vi "Chrg_Dschrg_nodaq.vi"(0 "Mod #":enum16{"0", "1", "2", "3"}(ring), 1 "Logical Instrument Number":u32=1, 3 "PS type":enum16{"ITECH", "NHR"}(ring), 4 "PS VISA in":refnum<visa-resource-name>, 5 "PS error in":errorcluster caption="PS error in (no error)", 6 "CyclePath":path=path "C:/Users/ga11/Desktop/VI/results/3PtestCharge.lvm" caption="Filename", 7 "Battery Type":T1(ring), 8 "Charge/discharge":enum8{"Charge", "Discharge"}(ring), 9 "Charge/Discharge Voltage Setpoint":dbl format="%#.6g", 11 "Current Setpoint":dbl format="%#.6g", 13 "Current Cutoff":dbl) -> (14 "PS VISA out":refnum<visa-resource-name>, 19 "PS error out":errorcluster)   [LabVIEW 2020]
uses:
  vi.lib/Utility/TradDaqScaling.llb/Convert Strain Gauge Reading (scaler).vi
  Drivers-NHR-9200/NHR/Public/Data/Read (Ave Current).vi
  Drivers-NHR-9200/NHR/Public/Data/Low Level/Fetch (Ave Voltage).vi
  Drivers-Essentials/NH Research Regenerative Test Series.lvlib
  Drivers-IT-M3400/IT-M3400.lvlib
panel:
  out "StrainGauge 2":dbl format="%.10f"
  out "Thermocouple 2":dbl format="%.2f"
  out "StrainGauge 1":dbl format="%.10f"
  out "Thermocouple 1":dbl format="%.2f"
  out "StrainGauge 3":dbl format="%.10f"
  out "Thermocouple 3":dbl format="%.2f"
  out "StrainGauge":dbl format="%.10f"
  out "Thermocouple":dbl format="%.2f"
  out "Read Ave Current (A)":dbl
  out "Read Ave Voltage (V)":dbl
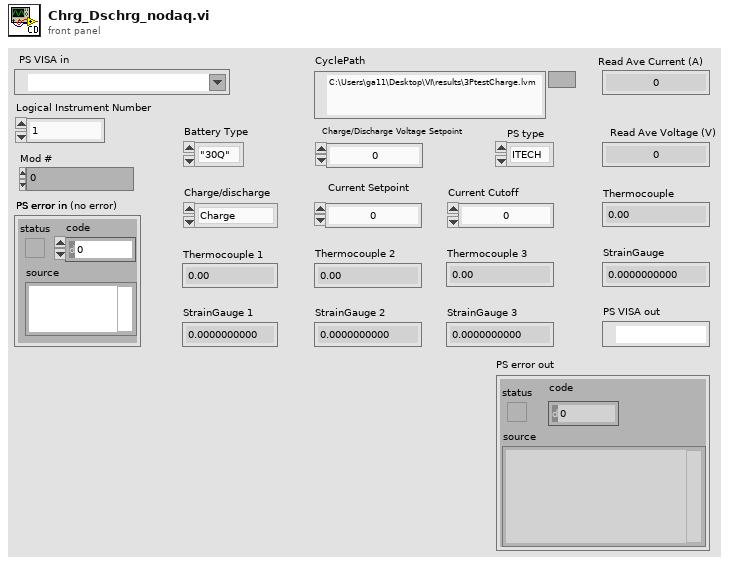
[diagram p1: front panel]
types:
  T1 = enum16{"\"30Q\"", "\"40T\"", "\"2P30Q\"", "\"3P30Q\"", "\"Nissan Leaf\""}
  T2 = cluster{"Min Voltage (V)":dbl, "Min Voltage Time (s)":dbl, "Max Voltage (V)":dbl, "Max Voltage Time (s)":dbl, "Max Sink Current (A)":dbl, "Max Sink Current Time (s)":dbl, "Max Source Current (A)":dbl, "Max Source Current Time (s)":dbl, "Max Sink Power (W)":dbl, "Max Sink Power Time (s)":dbl, "Max Source Power (W)":dbl, "Max Source Power Time (s)":dbl}
  T3 = cluster{"Voltage Enabled":bool, "Current Enabled":bool, "Power Enabled":bool, "Resistance Enabled":bool}
  T4 = cluster{"Baud Rate":u32, "Parity":u16, "Data Bits":u16, "Stop Bits":u16, "Flow Control":u16}
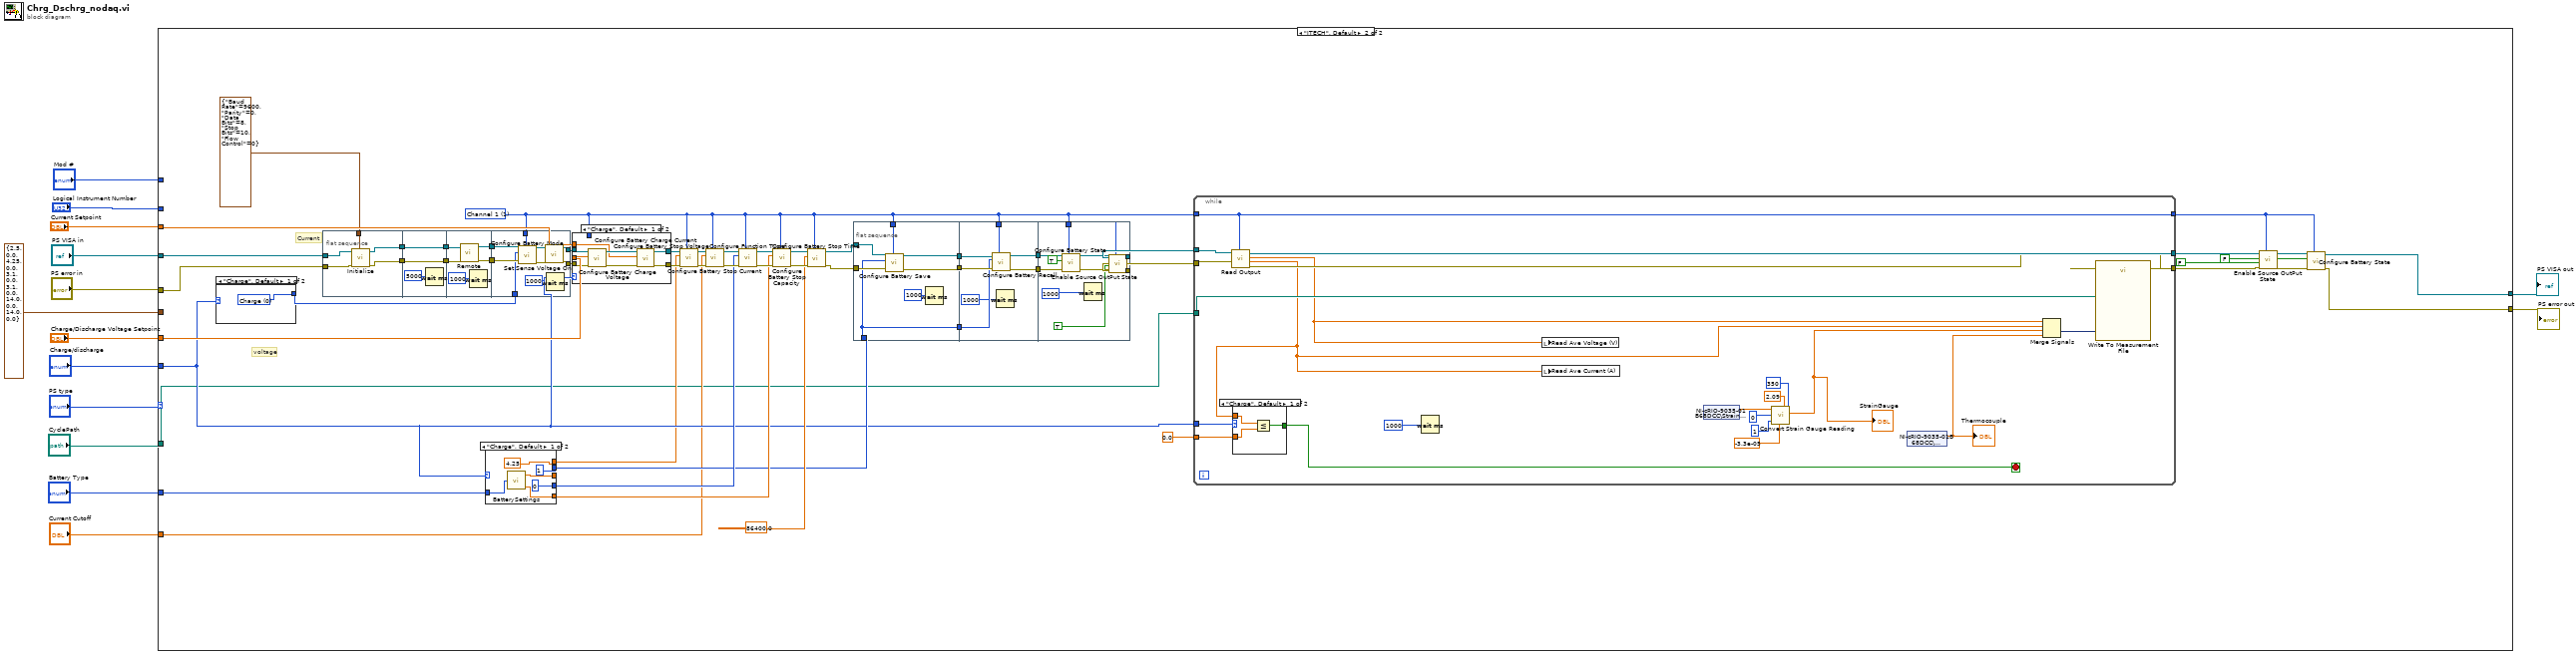
[diagram p0: block diagram]
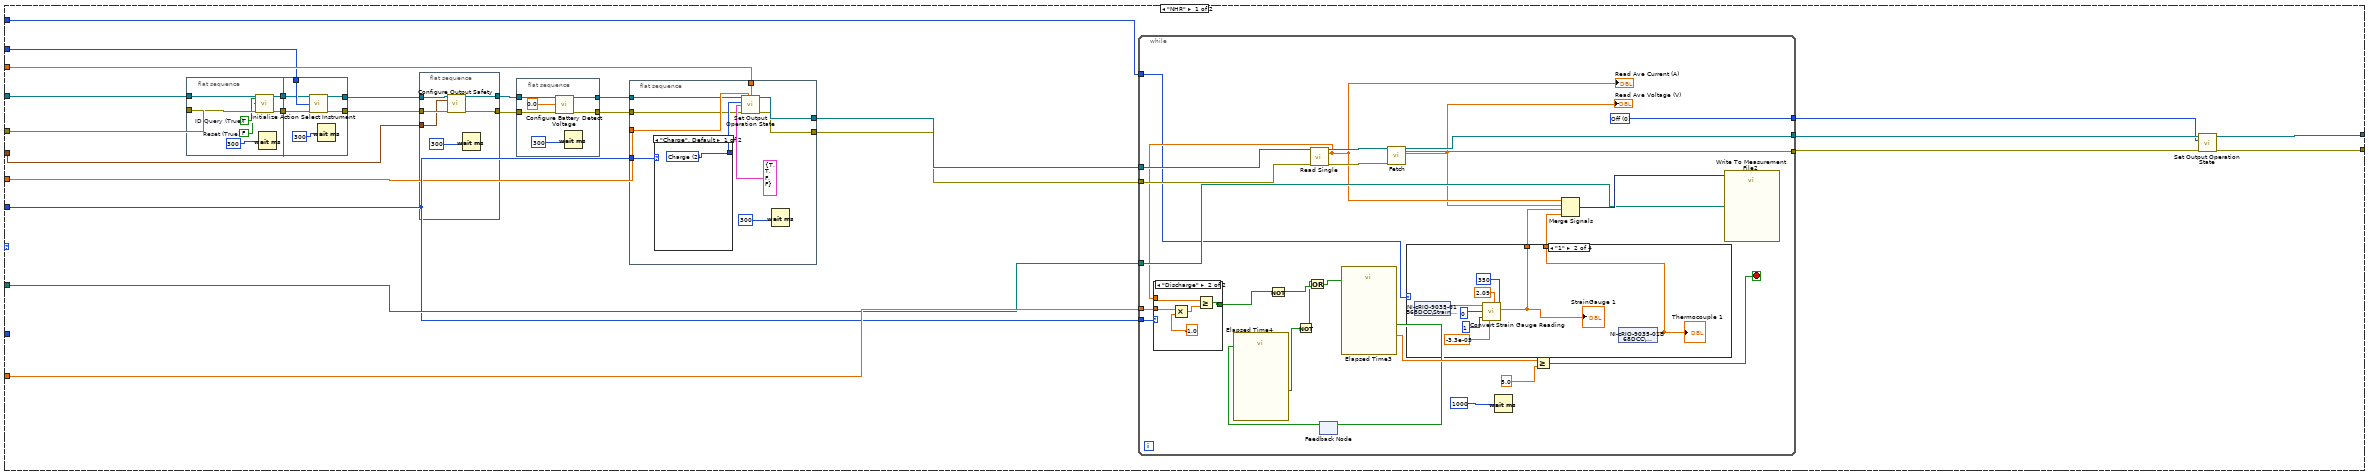
[diagram p2: hidden frame]
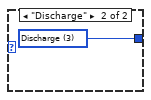
[diagram p3: hidden frame]
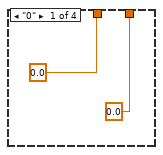
[diagram p4: hidden frame]
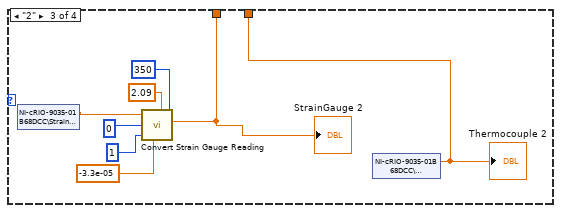
[diagram p5: hidden frame]
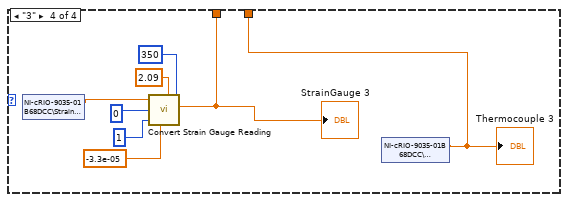
[diagram p6: hidden frame]
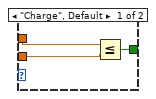
[diagram p7: hidden frame]
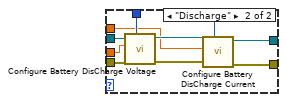
[diagram p8: hidden frame]
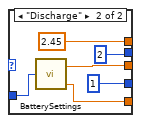
[diagram p9: hidden frame]
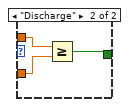
[diagram p10: hidden frame]
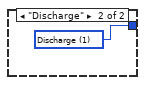
[diagram p11: hidden frame]
diagram:
  n1 = case shown="\"ITECH\", Default" "PS type" {
    tunnel: "Charge/Discharge Voltage Setpoint" -> [w29 w175]
    tunnel: "Current Setpoint" -> [w30 w173]
    tunnel: "Current Cutoff" -> [w37 w143]
    tunnel: "CyclePath" -> [w36 w141]
    tunnel: "PS VISA in" -> [w21 w154]
    tunnel: "PS error in" -> [w20 w153]
    tunnel: [w35 w140] -> w4
    tunnel: [w34 w174] -> w8
    tunnel: "Charge/discharge" -> [w31 w144]
    tunnel: "Battery Type" -> [_ w172]
    tunnel: "Mod #" -> [w27 _]
    tunnel: T2 {"Min Voltage (V)"=2.5, "Min Voltage Time (s)"=0.0, "Max Voltage (V)"=4.25, "Max Voltage Time (s)"=0.0, "Max Sink Current (A)"=3.1, "Max Sink Current Time (s)"=0.0, "Max Source Current (A)"=3.1, "Max Source Current Time (s)"=0.0, "Max Sink Power (W)"=14.0, "Max Sink Power Time (s)"=0.0, "Max Source Power (W)"=14.0, "Max Source Power Time (s)"=0.0} ("Output Safety") -> [w22 _]
    tunnel: "Logical Instrument Number" -> [w19 _]
    frame "NHR" {
      n2 = flat-sequence {
        tunnel: w21 -> [w46]
        tunnel: w20 -> [w45]
        tunnel: [w42] -> w16
        tunnel: [w41] -> w15
        tunnel: w19 -> [w52]
        tunnel: [w51] -> w18
        tunnel: [w50] -> w17
        tunnel: w16 -> [w49]
        tunnel: w15 -> [w48]
        frame #0 {
          w43 = FALSE  # Reset (True)
          w44 = TRUE  # ID Query (True)
          n3 = call "Initialize.vi"("VISA resource name"=w46, "ID Query (True)"=w44, "Reset (True)"=w43, "error in (no error)"=w45) -> ("VISA resource name out"=w41:refnum<visa-resource-name>, "error out"=w42:errorcluster)  [unwired: 10 in]
          n4 = Wait (ms)(milliseconds to wait=300) -> ()  [unwired: 1 out]
        }
        frame #1 {
          n5 = call "Action Select Instrument.vi"("VISA resource name"=w48, "Logical Instrument Number"=w52, "error in (no error)"=w49) -> ("VISA resource name out"=w51:refnum<visa-resource-name>, "error out"=w50:errorcluster)  [unwired: 11 in]
          n6 = Wait (ms)(milliseconds to wait=300) -> ()  [unwired: 1 out]
        }
      }
      n7 = flat-sequence {
        tunnel: w18 -> [w63]
        tunnel: w17 -> [w62]
        tunnel: [w61] -> w25
        tunnel: [w60] -> w26
        tunnel: w22 -> [w59]
        frame #0 {
          n8 = call "Configure Output Safety.vi"("VISA resource name"=w63, "Output Safety"=w59, "error in (no error)"=w62) -> ("VISA resource name out"=w60:refnum<visa-resource-name>, "error out"=w61:errorcluster)  [unwired: 11 in]
          n9 = Wait (ms)(milliseconds to wait=300) -> ()  [unwired: 1 out]
        }
      }
      n10 = flat-sequence {
        tunnel: w26 -> [w56]
        tunnel: w25 -> [w55]
        tunnel: [w54] -> w24
        tunnel: [w53] -> w23
        frame #0 {
          n11 = call "Configure Battery Detect Voltage.vi"("VISA resource name"=w56, "Battery Detect Voltage (0V)"=0.0, "error in (no error)"=w55) -> ("VISA resource name out"=w53:refnum<visa-resource-name>, "error out"=w54:errorcluster)  [unwired: 11 in]
          n12 = Wait (ms)(milliseconds to wait=300) -> ()  [unwired: 1 out]
        }
      }
      n13 = flat-sequence {
        tunnel: [w74] -> w39
        tunnel: [w73] -> w38
        tunnel: w31 -> [w71]
        tunnel: w30 -> [w70]
        tunnel: w29 -> [w69]
        tunnel: w24 -> [w66]
        tunnel: w23 -> [w65]
        frame #0 {
          n14 = case shown="\"Charge\", Default" w71 {
            tunnel: [w75 w76] -> w72
            frame "Charge", Default {
              w75 = 2 items=["Off", "Standby", "Charge", "Discharge", "Battery"] ("Mode (0: Off)")
            }
            frame "Discharge" {
              w76 = 3 items=["Off", "Standby", "Charge", "Discharge", "Battery"] ("Mode (0: Off)")
            }
          }
          n15 = call "Set Output Operation State.vi"("VISA resource name"=w65, "Voltage Setpoint (0 V)"=w69, "Current Setpoint (0 A)"=w70, "Mode (0: Off)"=w72, "Enable"=T3 {"Voltage Enabled"=TRUE, "Current Enabled"=TRUE, "Power Enabled"=FALSE, "Resistance Enabled"=FALSE}, "error in (no error)"=w66, "Power Setpoint (0 W)"=w69) -> ("VISA resource name out"=w74:refnum<visa-resource-name>, "error out"=w73:errorcluster)  [unwired: 7 in]
          n16 = Wait (ms)(milliseconds to wait=300) -> ()  [unwired: 1 out]
        }
      }
      n17 = while {
        tunnel: w39 -> [w101]
        tunnel: w38 -> [w100]
        tunnel: w37 -> [w85]
        tunnel: w36 -> [w88]
        tunnel: [w87] -> w33
        tunnel: [w86] -> w32
        tunnel: w31 -> [w84]
        tunnel: w27 -> [w78]
        tunnel: [w77] -> w28
        stop <- w91 stop-if-true
        w77 = 0 items=["Off", "Standby", "Charge", "Discharge", "Battery"] ("Mode (0: Off)")
        n18 = call-poly "Read Single.vi"("VISA resource name"=w101, "error in (no error)"=w100) -> ("VISA resource name out"=w102:refnum<visa-resource-name>, "Ave Current (A)"=w83:dbl, "error out"=w103:errorcluster)  [unwired: 11 in]
        "Read Ave Current (A)" <- w83
        n19 = case shown="\"Discharge\"" w84 {
          tunnel: w85 -> [w130 w136]
          tunnel: w83 -> [w132 w134]
          tunnel: [w131 w133] -> w82
          frame "Charge", Default {
            n20 = Less Or Equal?(x=w132, y=w130) -> (x <= y?=w131:bool)
          }
          frame "Discharge" {
            n21 = Multiply(x=w136, y=-1.0) -> (x*y=w135:dbl)
            n22 = Greater Or Equal?(x=w134, y=w135) -> (x >= y?=w133:bool)
          }
        }
        n23 = Not(x=w82) -> (.not. x?=w97:bool)
        n24 = feedback #1() -> (w89:bool)  [unwired: 1 in]
        n25 = call "Elapsed Time4"("Reset"=w89) -> ("Time has Elapsed"=w96:bool)  [unwired: 11 in, 7 out]
        n26 = Not(x=w96) -> (.not. x?=w95:bool)
        n27 = Or(x=w95, y=w97) -> (x .or. y?=w94:bool)
        n28 = call "Elapsed Time3"("Reset"=w94) -> ("Elapsed Time (s)"=w93:dbl, "Time has Elapsed"=w90:bool)  [unwired: 11 in, 6 out]
        n29 = feedback-in #1(w90) -> ()
        n30 = call-poly "Fetch.vi"("VISA resource name"=w102, "error in (no error)"=w103) -> ("VISA resource name out"=w87:refnum<visa-resource-name>, "Ave Voltage (V)"=w81:dbl, "error out"=w86:errorcluster)  [unwired: 11 in]
        "Read Ave Voltage (V)" <- w81
        n31 = case shown="\"1\"" w78 {
          tunnel: [0.0 w107 w116 w124] -> w80
          tunnel: [0.0 w106 w114 w123] -> w79
          frame "0" {
          }
          frame "1" {
            n32 = shared-variable "NI-cRIO-9035-01B68DCC\\Strain Gauge\\AI0"() -> (w108:dbl)  [unwired: 1 in, 1 out]
            n33 = call-poly "Convert Strain Gauge Reading.vi"("Vsg (0.0)"=w108, "Bridge Configuration\n(3:Half Bridge II)"=0, "Vex (3.33)"=1, "Vinit (0.0)"=-3.3e-05, "GF (2.0)"=2.09, "Rg (120)"=350) -> ("Strain"=w107:sgl)  [unwired: 4 in]
            "StrainGauge 1" <- w107
            n34 = shared-variable "NI-cRIO-9035-01B68DCC\\Thermocouple\\CH0"() -> (w106:dbl)  [unwired: 1 in, 1 out]
            "Thermocouple 1" <- w106
          }
          frame "2" {
            n35 = shared-variable "NI-cRIO-9035-01B68DCC\\Strain Gauge\\AI1"() -> (w115:dbl)  [unwired: 1 in, 1 out]
            n36 = call-poly "Convert Strain Gauge Reading.vi"("Vsg (0.0)"=w115, "Bridge Configuration\n(3:Half Bridge II)"=0, "Vex (3.33)"=1, "Vinit (0.0)"=-3.3e-05, "GF (2.0)"=2.09, "Rg (120)"=350) -> ("Strain"=w116:sgl)  [unwired: 4 in]
            "StrainGauge 2" <- w116
            n37 = shared-variable "NI-cRIO-9035-01B68DCC\\Thermocouple\\CH1"() -> (w114:dbl)  [unwired: 1 in, 1 out]
            "Thermocouple 2" <- w114
          }
          frame "3" {
            n38 = shared-variable "NI-cRIO-9035-01B68DCC\\Strain Gauge\\AI2"() -> (w122:dbl)  [unwired: 1 in, 1 out]
            n39 = call-poly "Convert Strain Gauge Reading.vi"("Vsg (0.0)"=w122, "Bridge Configuration\n(3:Half Bridge II)"=0, "Vex (3.33)"=1, "Vinit (0.0)"=-3.3e-05, "GF (2.0)"=2.09, "Rg (120)"=350) -> ("Strain"=w124:sgl)  [unwired: 4 in]
            "StrainGauge 3" <- w124
            n40 = shared-variable "NI-cRIO-9035-01B68DCC\\Thermocouple\\CH2"() -> (w123:dbl)  [unwired: 1 in, 1 out]
            "Thermocouple 3" <- w123
          }
        }
        n41 = Wait (ms)(milliseconds to wait=1000) -> ()  [unwired: 1 out]
        n42 = Greater Or Equal?(x=w93, y=5.0) -> (x >= y?=w91:bool)
        n43 = Merge Signals "Merge Signals"(w83, w81, w80, w79) -> (w99:dynamicdata)
        n44 = call "Write To Measurement File2"("Signals"=w99, "Filename"=w88) -> ()  [unwired: 15 in, 3 out]
      }
      n45 = call "Set Output Operation State.vi"("VISA resource name"=w33, "Mode (0: Off)"=w28, "error in (no error)"=w32) -> ("VISA resource name out"=w35:refnum<visa-resource-name>, "error out"=w34:errorcluster)  [unwired: 11 in]
    }
    frame "ITECH", Default {
      w146 = 1 items=["Channel 1"=1, "Channel 2"=2, "Channel 3"=3, "Channel 4"=4, "Channel 5"=5, "Channel 6"=6, "Channel 7"=7, "Channel 8"=8, "Channel 8"=9, "Channel 10"=10, "Channel 11"=11, "Channel 12"=12, "Channel 13"=13, "Channel 14"=14, "Channel 15"=15, "Channel 16"=16] ("Channel")
      # "voltage"
      # "Current"
      n46 = case shown="\"Charge\", Default" w144 {
        tunnel: [w293 w294] -> w160
        frame "Charge", Default {
          w293 = u8 0 items=["Charge", "Discharge"] ("Battery Mode")
        }
        frame "Discharge" {
          w294 = u8 1 items=["Charge", "Discharge"] ("Battery Mode")
        }
      }
      n47 = flat-sequence {
        tunnel: [w191] -> w158
        tunnel: [w192] -> w156
        tunnel: T4 {"Baud Rate"=9600, "Parity"=0, "Data Bits"=8, "Stop Bits"=10, "Flow Control"=0} ("Serial Configuration") -> [w195]
        tunnel: w153 -> [w194]
        tunnel: w154 -> [w193]
        tunnel: w158 -> [w198]
        tunnel: [w198] -> w157
        tunnel: w156 -> [w197]
        tunnel: [w197] -> w155
        tunnel: [w203] -> w162
        tunnel: [w202] -> w161
        tunnel: w157 -> [w201]
        tunnel: w155 -> [w200]
        tunnel: w162 -> [w209]
        tunnel: w161 -> [w211]
        tunnel: w146 -> [w212]
        tunnel: w160 -> [w210]
        tunnel: [w205] -> w139
        tunnel: [w204] -> w138
        frame #0 {
          n48 = call "Initialize.vi"("Serial Configuration"=w195, "error in"=w194, "VISA resource name"=w193) -> ("error out"=w192:errorcluster, "VISA resource name out"=w191:refnum<visa-resource-name>)  [unwired: 7 in]
        }
        frame #1 {
          n49 = Wait (ms)(milliseconds to wait=5000) -> ()  [unwired: 1 out]
        }
        frame #2 {
          n50 = call "Remote.vi"("error in"=w200, "VISA resource name"=w201) -> ("error out"=w202:errorcluster, "VISA resource name out"=w203:refnum<visa-resource-name>)  [unwired: 8 in]
          n51 = Wait (ms)(milliseconds to wait=1000) -> ()  [unwired: 1 out]
        }
        frame #3 {
          n52 = call "Configure Battery Mode.vi"("Channel"=w212, "error in"=w211, "Battery Mode"=w210, "VISA resource name"=w209) -> ("error out"=w206:errorcluster, "VISA resource name out"=w207:refnum<visa-resource-name>)  [unwired: 6 in]
          n53 = call "Set Sense Voltage On.vi"("error in"=w206, "VISA resource name"=w207) -> ("error out"=w205:errorcluster, "VISA resource name out"=w204:refnum<visa-resource-name>)  [unwired: 8 in]
          n54 = Wait (ms)(milliseconds to wait=1000) -> ()  [unwired: 1 out]
        }
      }
      n55 = case shown="\"Charge\", Default" w144 {
        tunnel: w172 -> [w259 w265]
        tunnel: [w258 w263] -> _
        tunnel: [u8 0 ("File") u8 1 ("File")] -> w148
        tunnel: [u8 1 ("File") u8 2 ("File")] -> w145
        tunnel: [w255 w261] -> w147
        tunnel: [4.25 2.45] -> w142
        frame "Charge", Default {
          n56 = call "BatterySettings.vi"("Battery Type"=w259) -> ("RatedCapacity (Ah)"=w255:dbl, "Max Voltage (V)"=w258:dbl)  [unwired: 2 in, 1 out]
        }
        frame "Discharge" {
          n57 = call "BatterySettings.vi"("Battery Type"=w265) -> ("RatedCapacity (Ah)"=w261:dbl, "Min Voltage (V)"=w263:dbl)  [unwired: 2 in, 1 out]
        }
      }
      n58 = case shown="\"Charge\", Default" w144 {
        tunnel: w138 -> [w244 w253]
        tunnel: w139 -> [w243 w252]
        tunnel: [w238 w249] -> w182
        tunnel: [w237 w248] -> w181
        tunnel: w146 -> [_ w247]
        tunnel: w175 -> [w240 w246]
        tunnel: w173 -> [w239 w245]
        frame "Charge", Default {
          n59 = call "Configure Battery Charge Voltage.vi"("error in"=w243, "Charge Voltage(V)"=w240, "VISA resource name"=w244) -> ("error out"=w241:errorcluster, "VISA resource name out"=w242:refnum<visa-resource-name>)  [unwired: 6 in]
          n60 = call "Configure Battery Charge Current.vi"("error in"=w241, "Charge Current(A)"=w239, "VISA resource name"=w242) -> ("error out"=w237:errorcluster, "VISA resource name out"=w238:refnum<visa-resource-name>)  [unwired: 7 in]
        }
        frame "Discharge" {
          n61 = call "Configure Battery DisCharge Voltage.vi"("Channel"=w247, "error in"=w252, "Discharge Voltage(V)"=w246, "VISA resource name"=w253) -> ("error out"=w250:errorcluster, "VISA resource name out"=w251:refnum<visa-resource-name>)  [unwired: 6 in]
          n62 = call "Configure Battery DisCharge Current.vi"("Channel"=w247, "error in"=w250, "Discharge Current(A)"=w245, "VISA resource name"=w251) -> ("error out"=w248:errorcluster, "VISA resource name out"=w249:refnum<visa-resource-name>)  [unwired: 6 in]
        }
      }
      n63 = call "Configure Battery Stop Voltage.vi"("Channel"=w146, "error in"=w181, "Stop Voltage(V)"=w142, "VISA resource name"=w182) -> ("error out"=w189:errorcluster, "VISA resource name out"=w190:refnum<visa-resource-name>)  [unwired: 6 in]
      n64 = call "Configure Battery Stop Current.vi"("Channel"=w146, "error in"=w189, "Stop Current(A)"=w143, "VISA resource name"=w190) -> ("error out"=w150:errorcluster, "VISA resource name out"=w152:refnum<visa-resource-name>)  [unwired: 6 in]
      n65 = call "Configure Function Type.vi"("Channel"=w146, "error in"=w150, "Function Type"=w148, "VISA resource name"=w152) -> ("error out"=w149:errorcluster, "VISA resource name out"=w151:refnum<visa-resource-name>)  [unwired: 6 in]
      n66 = call "Configure Battery Stop Capacity.vi"("Channel"=w146, "error in"=w149, "Stop Capacity(Ah)"=w147, "VISA resource name"=w151) -> ("error out"=w187:errorcluster, "VISA resource name out"=w188:refnum<visa-resource-name>)  [unwired: 6 in]
      n67 = call "Configure Battery Stop Time.vi"("Channel"=w146, "error in"=w187, "Stop Time(S)"=86400.0, "VISA resource name"=w188) -> ("error out"=w164:errorcluster, "VISA resource name out"=w163:refnum<visa-resource-name>)  [unwired: 6 in]
      n68 = flat-sequence {
        tunnel: w145 -> [w218]
        tunnel: w146 -> [w213]
        tunnel: [w216] -> w167
        tunnel: [w218] -> w166
        tunnel: [w215] -> w165
        tunnel: w164 -> [w219]
        tunnel: w163 -> [w217]
        tunnel: [w222] -> w169
        tunnel: [w223] -> w168
        tunnel: w167 -> [w226]
        tunnel: w166 -> [w225]
        tunnel: w165 -> [w224]
        tunnel: w146 -> [w220]
        tunnel: [w230] -> w180
        tunnel: [w229] -> w179
        tunnel: w146 -> [w228]
        tunnel: w169 -> [w236]
        tunnel: w168 -> [w235]
        frame #0 {
          n69 = call "Configure Battery Save.vi"("Channel"=w213, "error in"=w219, "File"=w218, "VISA resource name"=w217) -> ("error out"=w216:errorcluster, "VISA resource name out"=w215:refnum<visa-resource-name>)  [unwired: 6 in]
          n70 = Wait (ms)(milliseconds to wait=1000) -> ()  [unwired: 1 out]
        }
        frame #1 {
          n71 = call "Configure Battery Recall.vi"("Channel"=w220, "error in"=w226, "File"=w225, "VISA resource name"=w224) -> ("error out"=w223:errorcluster, "VISA resource name out"=w222:refnum<visa-resource-name>)  [unwired: 6 in]
          n72 = Wait (ms)(milliseconds to wait=1000) -> ()  [unwired: 1 out]
        }
        frame #2 {
          n73 = call "Configure Battery State.vi"("Channel"=w228, "error in"=w235, "State"=TRUE, "VISA resource name"=w236) -> ("error out"=w233:errorcluster, "VISA resource name out"=w234:refnum<visa-resource-name>)  [unwired: 6 in]
          n74 = Wait (ms)(milliseconds to wait=1000) -> ()  [unwired: 1 out]
          n75 = call "Enable Source OutPut State.vi"("Channel"=w228, "error in"=w233, "State"=TRUE ("Enable Output|Intput"), "VISA resource name"=w234) -> ("error out"=w229:errorcluster, "VISA resource name out"=w230:refnum<visa-resource-name>)  [unwired: 6 in]
        }
      }
      n76 = while {
        tunnel: [w278] -> w178
        tunnel: [w271] -> w177
        tunnel: w180 -> [w286]
        tunnel: w179 -> [w285]
        tunnel: w146 -> [w277]
        tunnel: [w277] -> w176
        tunnel: w141 -> [w283]
        tunnel: 0.0 -> [w281]
        tunnel: w144 -> [w279]
        stop <- w280 stop-if-true
        n77 = call "Read Output.vi"("Channel"=w277, "error in"=w285, "VISA resource name"=w286) -> ("error out"=w271:errorcluster, "Read Current(A)"=w269:dbl, "Read Voltage(V)"=w270:dbl, "VISA resource name out"=w278:refnum<visa-resource-name>)  [unwired: 5 in]
        n78 = case shown="\"Charge\", Default" w279 {
          tunnel: w281 -> [w288 w291]
          tunnel: w269 -> [w289 w292]
          tunnel: [w287 w290] -> w280
          frame "Charge", Default {
            n79 = Less Or Equal?(x=w289, y=w288) -> (x <= y?=w287:bool)
          }
          frame "Discharge" {
            n80 = Greater Or Equal?(x=w292, y=w291) -> (x >= y?=w290:bool)
          }
        }
        n81 = Wait (ms)(milliseconds to wait=1000) -> ()  [unwired: 1 out]
        n82 = local write "Read Ave Voltage (V)"(w270) -> ()
        n83 = local write "Read Ave Current (A)"(w269) -> ()
        n84 = shared-variable "NI-cRIO-9035-01B68DCC\\Strain Gauge\\AI0"() -> (w266:dbl)  [unwired: 1 in, 1 out]
        n85 = call-poly "Convert Strain Gauge Reading.vi"("Vsg (0.0)"=w266, "Bridge Configuration\n(3:Half Bridge II)"=0, "Vex (3.33)"=1, "Vinit (0.0)"=-3.3e-05, "GF (2.0)"=2.09, "Rg (120)"=350) -> ("Strain"=w268:sgl)  [unwired: 4 in]
        "StrainGauge" <- w268
        n86 = shared-variable "NI-cRIO-9035-01B68DCC\\Thermocouple\\CH0"() -> (w267:dbl)  [unwired: 1 in, 1 out]
        "Thermocouple" <- w267
        n87 = Merge Signals "Merge Signals"(w270, w269, w268, w267) -> (w284:dynamicdata)
        n88 = call "Write To Measurement File"("Signals"=w284, "Filename"=w283) -> ()  [unwired: 15 in, 3 out]
      }
      n89 = call "Enable Source OutPut State.vi"("Channel"=w176, "error in"=w177, "State"=FALSE, "VISA resource name"=w178) -> ("error out"=w185:errorcluster, "VISA resource name out"=w186:refnum<visa-resource-name>)  [unwired: 6 in]
      n90 = call "Configure Battery State.vi"("Channel"=w176, "error in"=w185, "State"=FALSE, "VISA resource name"=w186) -> ("error out"=w174:errorcluster, "VISA resource name out"=w140:refnum<visa-resource-name>)  [unwired: 6 in]
    }
  }
  "PS error out" <- w8
  "PS VISA out" <- w4
